vi "ReadDOs.vi"(8 "error in":errorcluster, 10 "Output":T1, 11 "VISA resource name":refnum<visa-resource-name>) -> (0 "error out":errorcluster, 2 "DO Status":bool, 3 "VISA resource name out":refnum<visa-resource-name>)   [LabVIEW 2020, in "HandsOnPi2040.lvlib"]
uses:
  HandsOnPi2040.lvlib
  DigOuts.ctl
  <vilib>/CTI/CTI Visa Drivers/CTI-Visa/CTI-Visa.lvlib
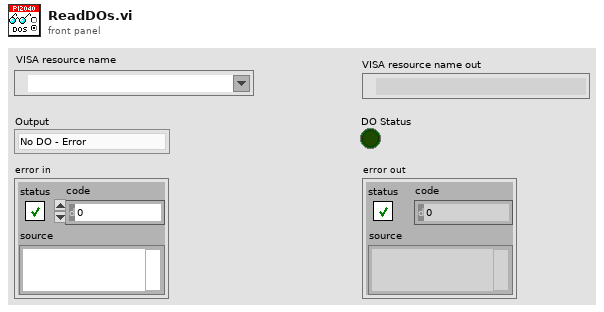
[diagram p1: front panel]
types:
  T1 = typedef "HandsOnPi2040.lvlib/DigOuts.ctl" = enum16{"No DO - Error", "DO1 (GPIO2)", "DO2 (GPIO3)", "DO3 (GPIO4)", "DO4 (GPIO5)", "BEEP (GPIO6)"}
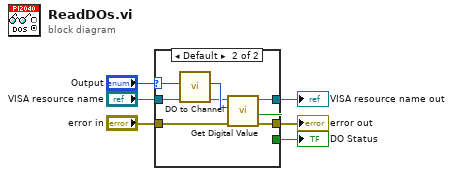
[diagram p0: block diagram]
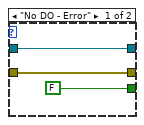
[diagram p2: hidden frame]
diagram:
  n1 = case shown="Default" "Output" {
    selector: "Output" -> [_ w10]
    tunnel: "VISA resource name" -> [w8 w13]
    tunnel: [w8 w12] -> w4
    tunnel: [w9 w15] -> w5
    tunnel: "error in" -> [w9 w16]
    tunnel: [FALSE ("Value") w11] -> w1
    frame "No DO - Error" {
    }
    frame Default {
      n2 = call "DO to Channel.vi"("Output"=w10) -> ("Channel"=w14:i32)  [unwired: 10 in]
      n3 = call <vilib>:"Get Digital Value.vi"("error in (no error)"=w16, "Channel"=w14, "VISA resource name in"=w13) -> ("error out"=w15:errorcluster, "Value"=w11:bool, "VISA resource name"=w12:refnum<visa-resource-name>)  [unwired: 6 in]
    }
  }
  "VISA resource name out" <- w4
  "DO Status" <- w1
  "error out" <- w5
